vi "DWF PS Query Tracking.vi"(0 "Instrument Handle In":u32, 11 "Error In":errorcluster caption="Error In (no error)") -> (4 "Instrument Handle Out":u32, 6 "Tracking Enabled":bool, 15 "Error Out":errorcluster)   [LabVIEW 2015, in "DigilentWF.lvlib"]
doc: "Indicates whether voltage tracking is enabled on the instrument."
uses:
  <vilib>/DigilentWF/DigilentWF.lvlib
  dwf.dll
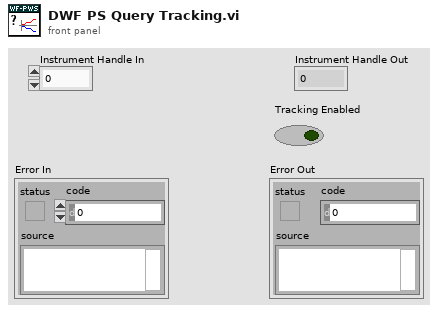
[diagram p1: front panel]
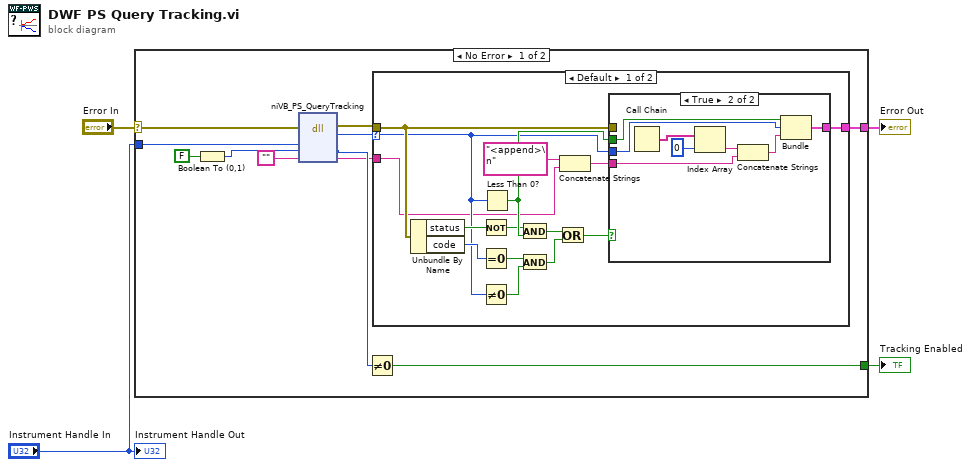
[diagram p0: block diagram]
diagram:
  n1 = case "outter_case" shown="No Error" "Error In" {
    selector: "Error In" -> [w12 w41]
    tunnel: [w15 w41] -> w3
    tunnel: "Instrument Handle In" -> [w11 _]
    tunnel: [w13 _] -> w1
    frame No Error {
      n2 = Boolean To (0,1)(Boolean=FALSE ("Tracking Enabled")) -> (0, 1=w10:i16)
      n3 = dll-call lib="dwf.*" fn="niVB_PS_QueryTracking"(error in=w12, "instrumentHandle"=w11, "trackingEnabled"=w10, "szError"="") -> (error out=w9:errorcluster, "return type"=w8:u32, "trackingEnabled"=w7:u32, "szError"=w5:string)  [unwired: 3 in, 1 out]
      n4 = Not Equal To 0?(x=w7) -> (x != 0?=w13:bool)
      n5 = case "inner_case" shown="Default" w8 {
        selector: w8 -> [w20 _]
        tunnel: w9 -> [w21 w40]
        tunnel: [w17 w40] -> w15
        tunnel: w5 -> [w16 _]
        frame Default {
          n6 = Unbundle By Name(w21) -> ("status"=w25:bool, "code"=w29:i32)
          n7 = Not(x=w25) -> (.not. x?=w28:bool)
          n8 = Equal To 0?(x=w29) -> (x = 0?=w24:bool)
          n9 = Not Equal To 0?(x=w20) -> (x != 0?=w27:bool)
          n10 = Less Than 0?(x=w20) -> (x < 0?=w30:bool)
          n11 = And(x=w28, y=w30) -> (x .and. y?=w26:bool)
          n12 = And(x=w24, y=w27) -> (x .and. y?=w23:bool)
          n13 = Or(x=w26, y=w23) -> (x .or. y?=w22:bool)
          n14 = Concatenate Strings("<append>\n" ("string"), w16) -> (w19:string)
          n15 = case shown="True" w22 {
            tunnel: [w31 w38] -> w17
            tunnel: w20 -> [_ w37]
            tunnel: w30 -> [_ w36]
            tunnel: w21 -> [w31 _]
            tunnel: w19 -> [_ w32]
            frame False {
            }
            frame True {
              n16 = Call Chain() -> (call chain=w35:string[])
              n17 = Index Array(array=w35, index=0) -> (element=w34:string)
              n18 = Concatenate Strings(w34, w32) -> (w39:string)
              n19 = Bundle(w36, "return type"=w37, w39) -> (w38:cluster{bool, "return type":u32, string})  [unwired: 1 out]
            }
          }
        }
        frame 0 {
        }
      }
    }
    frame Error {
    }
  }
  "Error Out" <- w3
  "Tracking Enabled" <- w1
  "Instrument Handle Out" <- "Instrument Handle In"
